vi "FITS hdr gen row by type.vi"(7 "Type":enum16{"String", "Integer", "Float"}(ring), 9 "Comment":string, 10 "Value":string, 11 "Header Field":string(combo)) -> (3 "FITS Row":string)   [LabVIEW 2020]
uses:
  FITS hdr gen row str.vi
  FITS hdr gen row int.vi
  FITS hdr gen row dbl.vi
  FIT Util Make Row 80 characters.vi
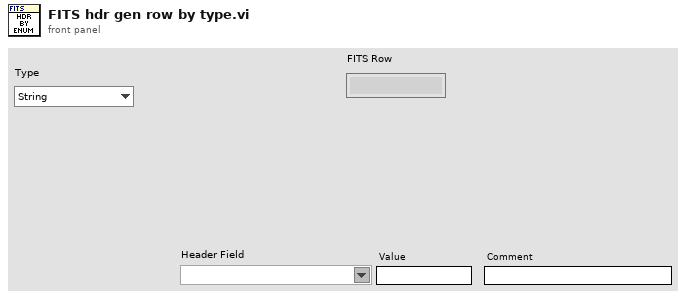
[diagram p1: front panel]
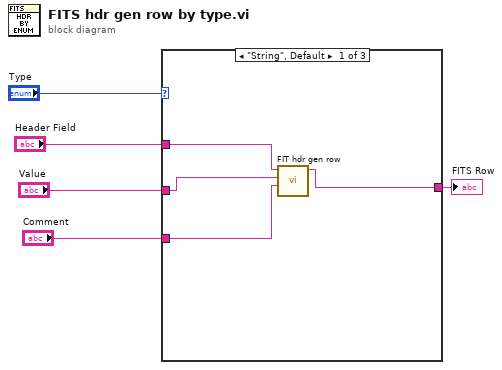
[diagram p0: block diagram]
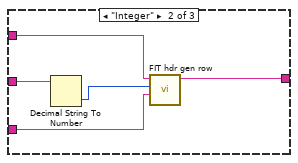
[diagram p2: hidden frame]
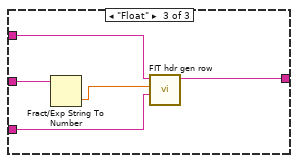
[diagram p3: hidden frame]
diagram:
  n1 = case shown="\"String\", Default" "Type" {
    tunnel: "Header Field" -> [w9 w12 w17]
    tunnel: "Value" -> [w8 w14 w19]
    tunnel: "Comment" -> [w7 w11 w16]
    tunnel: [w6 w10 w15] -> w1
    frame "String", Default {
      n2 = call-poly "FIT hdr gen row.vi"("Comment"=w7, "Value"=w8, "Field"=w9) -> ("FITS Row"=w6:string)  [unwired: 8 in]
    }
    frame "Integer" {
      n3 = Decimal String To Number(string=w14) -> (number=w13:i32)  [unwired: 2 in, 1 out]
      n4 = call-poly "FIT hdr gen row.vi"("Comment"=w11, "Value"=w13, "Field"=w12) -> ("FITS Row"=w10:string)  [unwired: 8 in]
    }
    frame "Float" {
      n5 = Fract/Exp String To Number(string=w19) -> (number=w18:dbl)  [unwired: 3 in, 1 out]
      n6 = call-poly "FIT hdr gen row.vi"("Comment"=w16, "Value"=w18, "Field"=w17) -> ("FITS Row"=w15:string)  [unwired: 8 in]
    }
  }
  "FITS Row" <- w1
